vi "GE 5565PIORC.Interrupts.Discard Events.vi"(8 "error in (no error)":errorcluster, 11 "GE 5565PIORC in":refnum<class "GE 5565PIORC.lvclass">) -> (0 "error out":errorcluster, 3 "GE 5565PIORC out":refnum<class "GE 5565PIORC.lvclass">)   [LabVIEW 2016, in "GE 5565PIORC.lvclass"]
doc: "Discards any events that may be pending for the PXI Interrupts used by the GE 5565PIORC."
uses:
  GE 5565PIORC.lvclass
  GE 5565PIORC.lvclass/GE 5565PIORC.ctl
  <vilib>/Instr/_visa.llb/Select Event Type.ctl
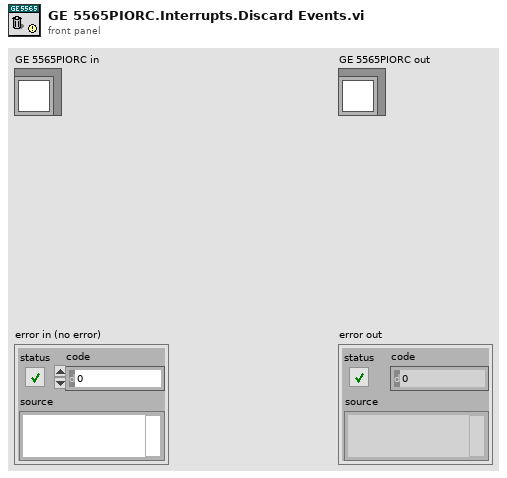
[diagram p1: front panel]
types:
  T1 = typedef "Select Event Type.ctl" = u32
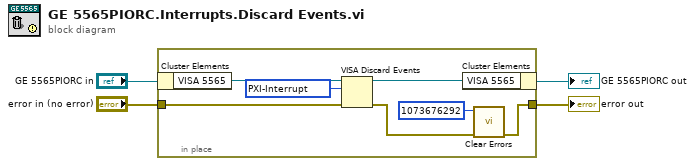
[diagram p0: block diagram]
diagram:
  n1 = in-place {
    in-place-border: "error in (no error)" -> [w6]
    in-place-border: [w5] -> w1
    w11 = T1 1073684514 items=["ServiceRequest"=1073684491, "Trigger"=3221168138, "Clear"=1073684493, "VXI-Signal"=1073684512, "VXI/VME-Interrupt"=3221168161, "VXI/VME-Sysfail"=1073684509, "VXI/VME-Sysreset"=1073684510, "GPIB-CIC"=1073684498, "GPIB-Talk"=1073684499, "GPIB-Listen"=1073684500, "PXI-Interrupt"=1073684514, "AllEnabled"=1073709055] ("Event Type")
    n2 = in-place-cluster #1("GE 5565PIORC in") -> ("VISA 5565"=w7:refnum<visa-resource-name>)
    n3 = VISA Discard Events(8:w6, 10:w11, 11:w7) -> (0:w9:errorcluster, 3:w8:refnum<visa-resource-name>)  [unwired: 1 in]
    n4 = in-place-cluster #1("VISA 5565"=w8) -> (→"GE 5565PIORC out":refnum<class "GE 5565PIORC.lvclass">)
    n5 = call <vilib>:"Clear Errors.vi"("error in (no error)"=w9, "specific error code to clear (0: all)"=1073676292) -> ("error out"=w5:errorcluster)  [unwired: 4 in, 1 out]
  }
  "error out" <- w1
